vi "GetPointsOnContour_combine.vi"(11 "origin contours":T2(array[cluster])) -> (2 "dinstance map":dbl[][](array[numeric]), 3 "check contours":T1(array[cluster]))   [LabVIEW 2017]
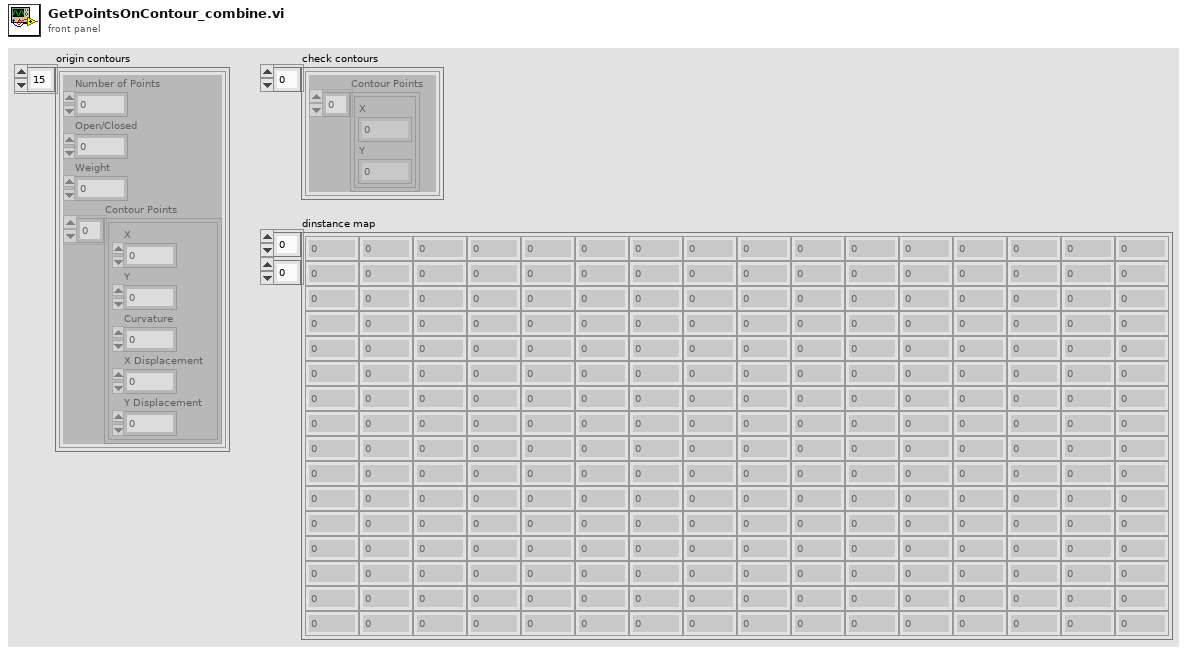
[diagram p1: front panel]
types:
  T1 = cluster{"Contour Points":cluster{"X":dbl, "Y":dbl}[]}[]
  T2 = cluster{"Number of Points":i32, "Open/Closed":i32, "Weight":dbl, "Contour Points":cluster{"X":dbl, "Y":dbl, "Curvature":dbl, "X Displacement":dbl, "Y Displacement":dbl}[]}[]
  T3 = cluster{"Number of Points":i32, "Open/Closed":i32, "Weight":dbl, "Contour Points":cluster{"X":dbl, "Y":dbl, "Curvature":dbl, "X Displacement":dbl, "Y Displacement":dbl}[]}
  T4 = cluster{"X":dbl, "Y":dbl, "Curvature":dbl, "X Displacement":dbl, "Y Displacement":dbl}[]
  T5 = cluster{"appended array":cluster{"X":dbl, "Y":dbl}[]}[]
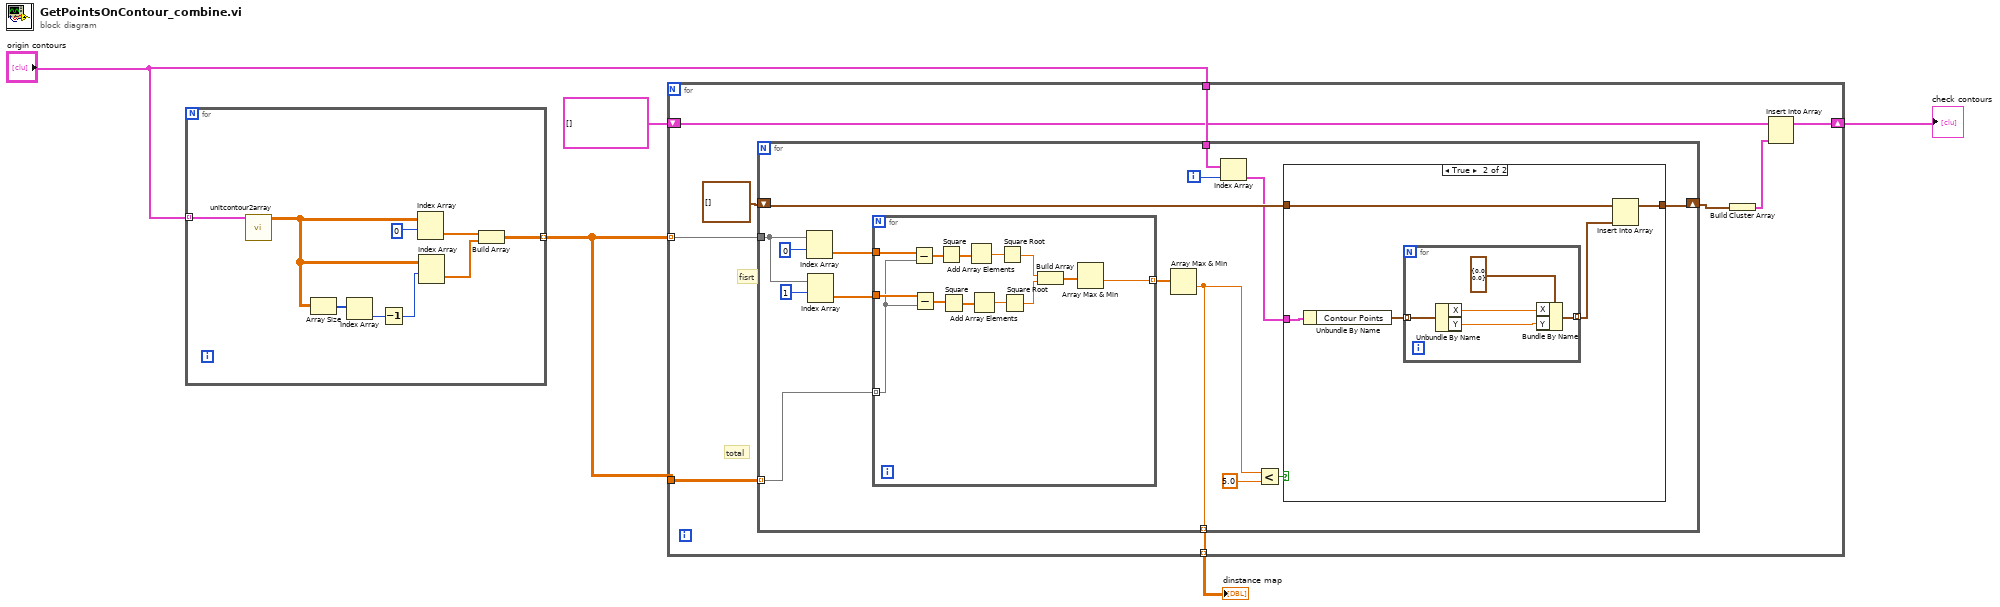
[diagram p0: block diagram]
diagram:
  n1 = for {
    tunnel: "origin contours" -> [w14] mode=indexing
    tunnel: [w6] -> w1 mode=indexing
    n2 = call "unitcontour2array.vi"("unit contour"=w14) -> ("Array"=w13:dbl[][])  [unwired: 10 in]
    n3 = Array Size(array=w13) -> (size(s)=w11:i32[])
    n4 = Index Array(array=w11) -> (element=w10:i32)  [unwired: 1 in]
    n5 = Decrement(x=w10) -> (x-1=w9:i32)
    n6 = Index Array(array=w13, index (row)=0) -> (element=w8:dbl[])  [unwired: 1 in]
    n7 = Index Array(array=w13, index (row)=w9) -> (element=w7:dbl[])  [unwired: 1 in]
    n8 = Build Array(w8, w7) -> (w6:dbl[][])
  }
  n9 = for {
    tunnel: w1 -> [w22] mode=indexing
    tunnel: w1 -> [w23]
    tunnel: [w21] -> w2 mode=indexing
    tunnel: "origin contours" -> [w19]
    shift-right: [w15] -> w5
    shift-left: T1 [] ("array of clusters") -> [w17]
    # "total"
    # "fisrt"
    n10 = for {
      tunnel: w23 -> [w33] mode=indexing
      tunnel: w22 -> [w36]
      tunnel: [w29] -> w21 mode=indexing
      shift-right: [w30] -> w18
      shift-left: cluster{"X":dbl, "Y":dbl}[] [] ("appended array") -> [w31]
      tunnel: w19 -> [w26]
      i -> [w24]
      n11 = Index Array(array=w36, index (row)=0) -> (element=w35:dbl[])  [unwired: 1 in]
      n12 = Index Array(array=w36, index (row)=1) -> (element=w34:dbl[])  [unwired: 1 in]
      n13 = for {
        tunnel: w35 -> [w62]
        tunnel: w34 -> [w61]
        tunnel: w33 -> [w60] mode=indexing
        tunnel: [w50] -> w32 mode=indexing
        n14 = Subtract(x=w62, y=w60) -> (x-y=w59:dbl[])
        n15 = Subtract(x=w61, y=w60) -> (x-y=w54:dbl[])
        n16 = Square(x=w59) -> (x^2=w57:dbl[])
        n17 = Square(x=w54) -> (x^2=w56:dbl[])
        n18 = Add Array Elements(numeric array=w57) -> (sum=w58:dbl)
        n19 = Add Array Elements(numeric array=w56) -> (sum=w55:dbl)
        n20 = Square Root(x=w58) -> (sqrt(x)=w53:dbl)
        n21 = Square Root(x=w55) -> (sqrt(x)=w52:dbl)
        n22 = Build Array(w53, w52) -> (w51:dbl[])
        n23 = Array Max & Min(array=w51) -> (min value=w50:dbl)  [unwired: 3 out]
      }
      n24 = Array Max & Min(array=w32) -> (min value=w29:dbl)  [unwired: 3 out]
      n25 = Index Array(array=w26, index=w24) -> (element=w25:T3)
      n26 = Less?(x=w29, y=5.0) -> (x < y?=w28:bool)
      n27 = case shown="True" w28 {
        tunnel: w31 -> [w39 w44]
        tunnel: w25 -> [_ w42]
        tunnel: [w39 w40] -> w30
        frame False {
        }
        frame True {
          n28 = Unbundle By Name(w42) -> ("Contour Points"=w43:T4)
          n29 = for {
            tunnel: w43 -> [w49] mode=indexing
            tunnel: [w45] -> w41 mode=indexing
            n30 = Unbundle By Name(w49) -> ("X"=w47:dbl, "Y"=w46:dbl)
            n31 = Bundle By Name(cluster=cluster{"X":dbl, "Y":dbl} {"X"=0.0, "Y"=0.0} ("Contour Point"), "X"=w47, "Y"=w46) -> (w45:cluster{"X":dbl, "Y":dbl})
          }
          n32 = Insert Into Array(array=w44, new element=w41) -> (w40:cluster{"X":dbl, "Y":dbl}[])  [unwired: 1 in]
        }
      }
    }
    n33 = Build Cluster Array(w18) -> (w16:T5)
    n34 = Insert Into Array(array=w17, new element=w16) -> (w15:T1)  [unwired: 1 in]
  }
  "dinstance map" <- w2
  "check contours" <- w5
